vi "主函数.vi"() -> ()   [LabVIEW 2020]
doc: "UDP协议与TCP的区别在于UDP不包括发送数据包信息的错误检查，因此无法保证接收端是否已接收所发数据。\n\nUDP可用于“广播”数据至整个网络，只需指定可包括全部的IP地址(255.255.255.255)以便发送信息至整个网络。 由于路由器或其他网络硬件通常拒绝转发超过一定点的数据，在实际应用中广播范围可能存在限制。"
panel:
  in  "停止输入":bool
  out "输出波形":waveform(i32)[](graph)
  in  "输出文件夹名称":path
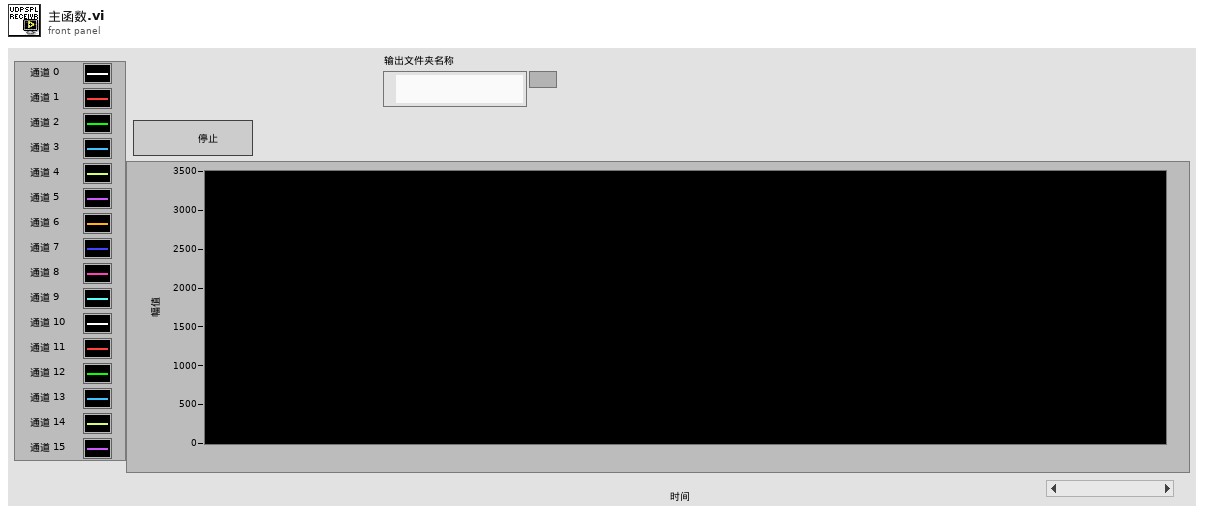
[diagram p1: front panel]
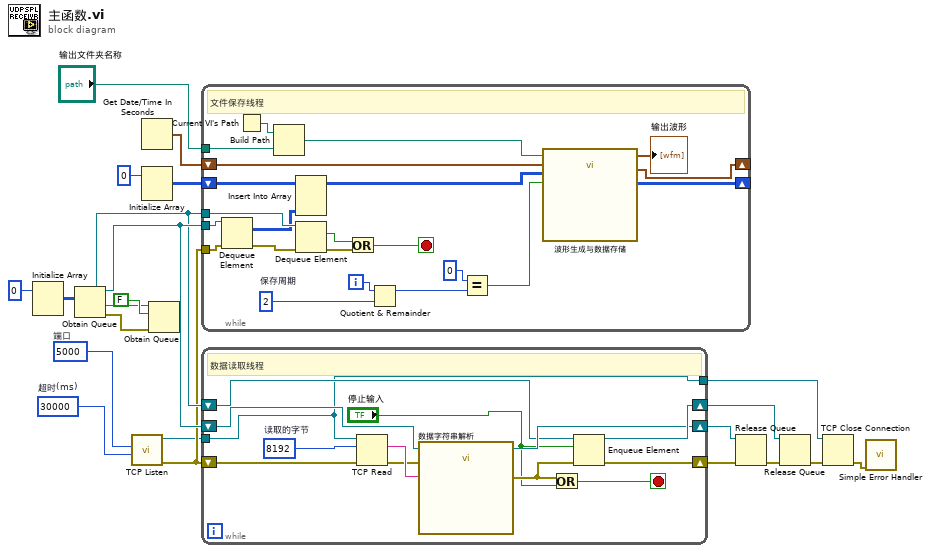
[diagram p0: block diagram]
diagram:
  w9 = 30000  # 超时(ms)
  w10 = u16 5000  # 端口
  n1 = Initialize Array(0) -> (w13:i32[][])  [unwired: 2 in]
  n2 = Obtain Queue(element data type=w13) -> (queue out=w7:refnum<queue>, error out=w14:errorcluster)  [unwired: 4 in, 1 out]
  n3 = call <vilib>:"TCP Listen.vi"("timeout ms (wait forever: -1)"=w9, "port"=w10) -> ("error out"=w5:errorcluster, "connection ID"=w4:refnum<k5>)  [unwired: 5 in, 3 out]
  n4 = Get Date/Time In Seconds() -> (seconds since 1Jan1904=w20:timestamp)
  n5 = Initialize Array(0) -> (w8:i32[][])  [unwired: 2 in]
  n6 = Obtain Queue(element data type=FALSE, error in (no error)=w14) -> (queue out=w6:refnum<queue>)  [unwired: 3 in, 2 out]
  n7 = while {
    tunnel: w5 -> [w43]
    tunnel: w7 -> [w41]
    tunnel: w6 -> [w39]
    shift-right: [w28] -> _
    shift-left: w8 -> [w35]
    shift-right: [w27] -> _
    shift-left: w20 -> [w26]
    tunnel: "输出文件夹名称" -> [w23]
    i -> [w34]
    stop <- w42 stop-if-true
    w33 = 2  # 保存周期
    # "文件保存线程"
    n8 = Dequeue Element(queue=w41, error in (no error)=w43) -> (element=w36:i32[][], error out=w40:errorcluster)  [unwired: 1 in, 2 out]
    n9 = Current VI's Path() -> (path=w25:path)
    n10 = Build Path(base path=w25, name or relative path=w23) -> (appended path=w24:path)
    n11 = Insert Into Array(array=w35, new element=w36) -> (w29:i32[][])  [unwired: 2 in]
    n12 = Dequeue Element(queue=w39, error in (no error)=w40) -> (element=w38:bool, error out=w37:errorcluster)  [unwired: 1 in, 2 out]
    n13 = Or(x=w38, y=w37) -> (x .or. y?=w42:bool)
    n14 = Quotient & Remainder(x=w34, y=w33) -> (x-y*floor(x/y)=w31:i32)  [unwired: 1 out]
    n15 = Equal?(x=0, y=w31) -> (x = y?=w30:bool)
    n16 = call "波形生成与数据存储.vi"("文件保存控制位"=w30, "数据输入"=w29, "上一时刻时间输入"=w26, "文件存储地址"=w24) -> ("缓存区输出"=w28:i32[][], "时间输出"=w27:timestamp, "输出波形"=→"输出波形":waveform(i32)[])  [unwired: 5 in]
  }
  n17 = while "While循环" {
    tunnel: w4 -> [w45]
    shift-right: [w53] -> w16
    shift-left: w5 -> [w47]
    shift-right: [w54] -> w17
    shift-left: w7 -> [w55]
    shift-right: [w56] -> w18
    shift-left: w6 -> [w50]
    tunnel: [w45] -> w3
    stop <- w51 stop-if-true
    w46 = 8192  # 读取的字节
    # "数据读取线程"
    n18 = TCP Read(connection ID=w45, bytes to read=w46, error in (no error)=w47) -> (data out=w49:string, error out=w48:errorcluster)  [unwired: 2 in, 1 out]
    n19 = call "数据字符串解析.vi"("输入数据"=w49, "错误输入（无错误）"=w48, "回传数据队列"=w55) -> ("错误输出"=w52:errorcluster, "回传数据队列"=w54:refnum<queue>)  [unwired: 7 in]
    n20 = Or(x=w52, y="停止输入") -> (x .or. y?=w51:bool)
    n21 = Enqueue Element(queue=w50, element="停止输入", error in (no error)=w52) -> (queue out=w56:refnum<queue>, error out=w53:errorcluster)  [unwired: 1 in, 1 out]
  }
  n22 = Release Queue(queue=w17, error in (no error)=w16) -> (error out=w19:errorcluster)  [unwired: 1 in, 2 out]
  n23 = Release Queue(queue=w18, error in (no error)=w19) -> (error out=w1:errorcluster)  [unwired: 1 in, 2 out]
  n24 = TCP Close Connection(connection ID=w3, error in (no error)=w1) -> (error out=w2:errorcluster)  [unwired: 1 in, 1 out]
  n25 = call <vilib>:"Simple Error Handler.vi"("error in (no error)"=w2) -> ()  [unwired: 4 in, 5 out]
